vi "Finish.vi"   [LabVIEW 2015]
doc: "This VI is called just before exiting. It is expected to close I/O refnum, save collected data, etc."
uses:
  <vilib>/Rock Robotics/WPI/Utilities/WPI_GetSetVariantRefNum.vi
types:
  T1 = typedef "WPI_JoystickDevRef.ctl" = cluster{"Device":T2}
  T2 = typedef "WPI_JoystickDeviceEnum.ctl" = enum16{"USB 0", "USB 1", "USB 2", "USB 3", "USB 4", "USB 5"}
  T3 = typedef "WPI_MotorControlDeviceRef.ctl" = cluster{"DeviceStatus":errorcluster, "Type":T4, "PWM":cluster{"PWM Channel":T5, "DeadBand":T6}, "CAN":cluster{"Device Number":u8, "Control Mode":T7, "Semaphore":T8, "Max Vout":dbl, "TalonSRX Control Mode":T9}, "Invert":bool}
  T4 = typedef "WPI_MotorControlType.ctl" = enum16{"PWM", "CAN", "CANTalonSRX"}
  T5 = typedef "FPGA_DIOPWMChannel.ctl" = enum8{"PWM 0", "PWM 1", "PWM 2", "PWM 3", "PWM 4", "PWM 5", "PWM 6", "PWM 7", "PWM 8", "PWM 9", "PWM MXP 0", "PWM MXP 1", "PWM MXP 2", "PWM MXP 3", "PWM MXP 4", "PWM MXP 5", "PWM MXP 6", "PWM MXP 7", "PWM MXP 8", "PWM MXP 9", "Invalid"}
  T6 = typedef "WPI_PWMDeadband.ctl" = cluster{"Name":string, "maxPositivePwm":i32, "minPositivePwm":i32, "centerPwm":i32, "maxNegativePwm":i32, "minNegativePwm":i32, "angularRange":u16}
  T7 = typedef "WPI_CANJaguar_ControlMode.ctl" = enum8{"Percent VBus", "Current", "Speed", "Position", "Voltage"}
  T8 = typedef "Semaphore RefNum" = refnum<k1>
  T9 = typedef "WPI_CANTalonSRX_APIControlMode.ctl" = enum8{"Percent VBus", "Speed", "Position", "Slave", "Unchanged / Invalid", "Voltage Compensation", "Current", "Motion Profile"}
  T10 = typedef "WPI_CompressorDevRef.ctl" = cluster{"DevStatus":errorcluster, "Pneumatics Control Module":u8}
  T11 = typedef "WPI_EncoderDevRef.ctl" = cluster{"DevStatus":errorcluster, "EncoderIndex":T12, "CounterIndex":T13, "DistancePerCount":dbl, "Decoding Type":T14}
  T12 = typedef "FPGA_EncoderIdx.ctl" = enum8{"Enc 0", "Enc 1", "Enc 2", "Enc 3", "Enc 4", "Enc 5", "Enc 6", "Enc 7", "Invalid"}
  T13 = typedef "FPGA_CounterCtrSystemIndex.ctl" = enum8{"Ctr 0", "Ctr 1", "Ctr 2", "Ctr 3", "Ctr 4", "Ctr 5", "Ctr 6", "Ctr 7", "Invalid"}
  T14 = typedef "WPI_EncoderType.ctl" = enum16{"1x", "2x", "4x"}
  T15 = typedef "WPI_SolenoidDevRef.ctl" = cluster{"DevStatus":errorcluster, "Pneumatics Control Module":u8, "Forward Solenoid Channel":T16, "Reverse Solenoid Channel":T16}
  T16 = typedef "WPI_SolenoidChannel.ctl" = enum8{"Solenoid 0", "Solenoid 1", "Solenoid 2", "Solenoid 3", "Solenoid 4", "Solenoid 5", "Solenoid 6", "Solenoid 7", "Invalid"}
  T17 = typedef "WPI_ServoDeviceRef.ctl" = cluster{"DeviceStatus":errorcluster, "PWM Channel":T5, "DeadBand":T6}
  T18 = typedef "WPI_SwitchDevRef.ctl" = cluster{"DevStatus":errorcluster, "DIO Channel":T19, "CntIndex":T13, "Normally Closed":bool}
  T19 = typedef "FPGA_DIOChannel.ctl" = enum8{"DIO 0", "DIO 1", "DIO 2", "DIO 3", "DIO 4", "DIO 5", "DIO 6", "DIO 7", "DIO 8", "DIO 9", "DIO MXP 0", "DIO MXP 1", "DIO MXP 2", "DIO MXP 3", "DIO MXP 4", "DIO MXP 5", "DIO MXP 6", "DIO MXP 7", "DIO MXP 8", "DIO MXP 9", "DIO MXP 10", "DIO MXP 11", "DIO MXP 12", "DIO MXP 13", "DIO MXP 14", "DIO MXP 15", "Invalid"}
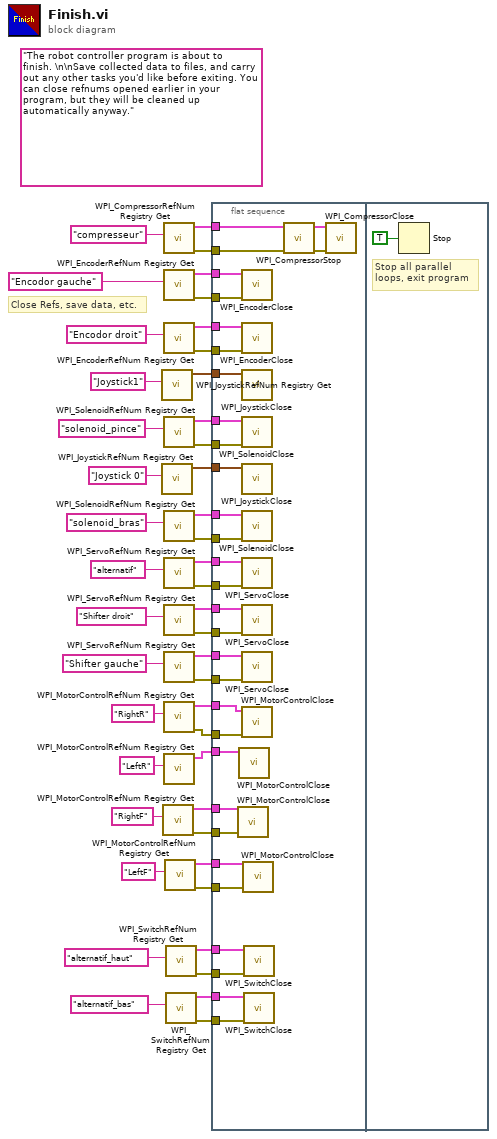
[diagram p0: block diagram]
diagram:
  (unwired) "The robot controller program is about to finish. \n\nSave collected data to files, and carry out any other tasks you'd like before exiting. You can close refnums opened earlier in your program, but they will be cleaned up automatically anyway."
  # "Close Refs, save data, etc."
  n1 = call <vilib>:"WPI_JoystickRefNum Registry Get.vi"("refnum name"="Joystick1") -> ("JoystickDevRef"=w32:T1)  [unwired: 1 in, 9 out]
  n2 = call <vilib>:"WPI_JoystickRefNum Registry Get.vi"("refnum name"="Joystick 0") -> ("JoystickDevRef"=w44:T1)  [unwired: 1 in, 9 out]
  n3 = call <vilib>:"WPI_MotorControlRefNum Registry Get.vi"("refnum name"="RightF") -> ("error out"=w6:errorcluster, "MotorControlDevRef"=w10:T3)  [unwired: 9 in]
  n4 = call <vilib>:"WPI_CompressorRefNum Registry Get.vi"("refnum name"="compresseur") -> ("error out"=w26:errorcluster, "CompressorDevRef"=w27:T10)  [unwired: 9 in]
  n5 = call <vilib>:"WPI_EncoderRefNum Registry Get.vi"("refnum name"="Encodor gauche") -> ("error out"=w21:errorcluster, "EncoderDevRef"=w22:T11)  [unwired: 9 in]
  n6 = call <vilib>:"WPI_EncoderRefNum Registry Get.vi"("refnum name"="Encodor droit") -> ("error out"=w20:errorcluster, "EncoderDevRef"=w19:T11)  [unwired: 9 in]
  n7 = call <vilib>:"WPI_SolenoidRefNum Registry Get.vi"("refnum name"="solenoid_pince") -> ("error out"=w18:errorcluster, "SolenoidDevRef"=w28:T15)  [unwired: 9 in]
  n8 = call <vilib>:"WPI_SolenoidRefNum Registry Get.vi"("refnum name"="solenoid_bras") -> ("error out"=w17:errorcluster, "SolenoidDevRef"=w31:T15)  [unwired: 9 in]
  n9 = call <vilib>:"WPI_ServoRefNum Registry Get.vi"("refnum name"="alternatif") -> ("error out"=w12:errorcluster, "ServoDeviceRef"=w38:T17)  [unwired: 9 in]
  n10 = call <vilib>:"WPI_ServoRefNum Registry Get.vi"("refnum name"="Shifter droit") -> ("error out"=w16:errorcluster, "ServoDeviceRef"=w43:T17)  [unwired: 9 in]
  n11 = call <vilib>:"WPI_ServoRefNum Registry Get.vi"("refnum name"="Shifter gauche") -> ("error out"=w15:errorcluster, "ServoDeviceRef"=w42:T17)  [unwired: 9 in]
  n12 = call <vilib>:"WPI_MotorControlRefNum Registry Get.vi"("refnum name"="RightR") -> ("error out"=w7:errorcluster, "MotorControlDevRef"=w8:T3)  [unwired: 9 in]
  n13 = call <vilib>:"WPI_MotorControlRefNum Registry Get.vi"("refnum name"="LeftR") -> ("MotorControlDevRef"=w9:T3)  [unwired: 9 in, 1 out]
  n14 = call <vilib>:"WPI_MotorControlRefNum Registry Get.vi"("refnum name"="LeftF") -> ("error out"=w5:errorcluster, "MotorControlDevRef"=w11:T3)  [unwired: 9 in]
  n15 = call <vilib>:"WPI_SwitchRefNum Registry Get.vi"("refnum name"="alternatif_haut") -> ("error out"=w13:errorcluster, "SwitchDevRef"=w35:T18)  [unwired: 9 in]
  n16 = call <vilib>:"WPI_SwitchRefNum Registry Get.vi"("refnum name"="alternatif_bas") -> ("error out"=w14:errorcluster, "SwitchDevRef"=w34:T18)  [unwired: 9 in]
  n17 = flat-sequence {
    tunnel: w44 -> [w76]
    tunnel: w43 -> [w75]
    tunnel: w42 -> [w74]
    tunnel: w38 -> [w73]
    tunnel: w35 -> [w72]
    tunnel: w34 -> [w71]
    tunnel: w32 -> [w70]
    tunnel: w31 -> [w69]
    tunnel: w28 -> [w68]
    tunnel: w27 -> [w65]
    tunnel: w26 -> [w64]
    tunnel: w22 -> [w63]
    tunnel: w21 -> [w62]
    tunnel: w20 -> [w61]
    tunnel: w19 -> [w60]
    tunnel: w18 -> [w59]
    tunnel: w17 -> [w58]
    tunnel: w16 -> [w57]
    tunnel: w15 -> [w56]
    tunnel: w14 -> [w55]
    tunnel: w13 -> [w54]
    tunnel: w12 -> [w53]
    tunnel: w11 -> [w52]
    tunnel: w10 -> [w51]
    tunnel: w9 -> [w50]
    tunnel: w8 -> [w49]
    tunnel: w7 -> [w48]
    tunnel: w6 -> [w47]
    tunnel: w5 -> [w46]
    frame #0 {
      n18 = call <vilib>:"WPI_MotorControlClose.vi"("error in (no error)"=w47, "MotorControlDevRef"=w51) -> ()  [unwired: 9 in, 1 out]
      n19 = call <vilib>:"WPI_MotorControlClose.vi"("MotorControlDevRef"=w50) -> ()  [unwired: 10 in, 1 out]
      n20 = call <vilib>:"WPI_EncoderClose.vi"("error in (no error)"=w62, "EncoderDevRef"=w63) -> ()  [unwired: 9 in, 1 out]
      n21 = call <vilib>:"WPI_EncoderClose.vi"("error in (no error)"=w61, "EncoderDevRef"=w60) -> ()  [unwired: 9 in, 1 out]
      n22 = call <vilib>:"WPI_JoystickClose.vi"("JoystickDevRef"=w70) -> ()  [unwired: 11 out]
      n23 = call <vilib>:"WPI_SolenoidClose.vi"("error in (no error)"=w59, "SolenoidDevRef"=w68) -> ()  [unwired: 9 in, 1 out]
      n24 = call <vilib>:"WPI_JoystickClose.vi"("JoystickDevRef"=w76) -> ()  [unwired: 11 out]
      n25 = call <vilib>:"WPI_SolenoidClose.vi"("error in (no error)"=w58, "SolenoidDevRef"=w69) -> ()  [unwired: 9 in, 1 out]
      n26 = call <vilib>:"WPI_ServoClose.vi"("error in (no error)"=w53, "ServoDeviceRef"=w73) -> ()  [unwired: 9 in, 1 out]
      n27 = call <vilib>:"WPI_ServoClose.vi"("error in (no error)"=w57, "ServoDeviceRef"=w75) -> ()  [unwired: 9 in, 1 out]
      n28 = call <vilib>:"WPI_ServoClose.vi"("error in (no error)"=w56, "ServoDeviceRef"=w74) -> ()  [unwired: 9 in, 1 out]
      n29 = call <vilib>:"WPI_MotorControlClose.vi"("error in (no error)"=w48, "MotorControlDevRef"=w49) -> ()  [unwired: 9 in, 1 out]
      n30 = call <vilib>:"WPI_MotorControlClose.vi"("error in (no error)"=w46, "MotorControlDevRef"=w52) -> ()  [unwired: 9 in, 1 out]
      n31 = call <vilib>:"WPI_SwitchClose.vi"("error in (no error)"=w54, "SwitchDevRef"=w72) -> ()  [unwired: 9 in, 1 out]
      n32 = call <vilib>:"WPI_SwitchClose.vi"("error in (no error)"=w55, "SwitchDevRef"=w71) -> ()  [unwired: 9 in, 1 out]
      n33 = call <vilib>:"WPI_CompressorStop.vi"("error in (no error)"=w64, "CompressorDevRef"=w65) -> ("error out"=w67:errorcluster, "CompressorDevRef"=w66:T10)  [unwired: 8 in]
      n34 = call <vilib>:"WPI_CompressorClose.vi"("error in (no error)"=w67, "CompressorDevRef"=w66) -> ()  [unwired: 9 in, 1 out]
    }
    frame #1 {
      # "Stop all parallel\nloops, exit program"
      n35 = Stop(stop? (T)=TRUE ("Quit")) -> ()
    }
  }
